vi "DailyReportSelectFromDateToDate.vi"() -> ()   [LabVIEW 2012]
uses:
  <vilib>/Utility/NIReport.llb/NI_report.lvclass
  Global1.vi
  <vilib>/Utility/NIReport.llb/Append Text Table to Report (wrap).vi
  <vilib>/Utility/NIReport.llb/Excel/NI_Excel.lvclass
  <vilib>/addons/_office/NI_ReportGenerationToolkit.lvlib
panel:
  in  "OK Button":bool
  in  "stop":bool
  in  "From Date (起日)":string="2014/9/20"
  in  "End Date (ùら)":string="2014/9/24"
  out "error out":errorcluster
  in  "ShiftB":string[][](array[string])
  in  "ShiftA":string[][](array[string])
  in  "ShiftC":string[][](array[string])
  in  "Summary":string[][](array[string])
  out "Row Headers":string[](array[string])
  in  "MonthToDate":string[][](array[string])
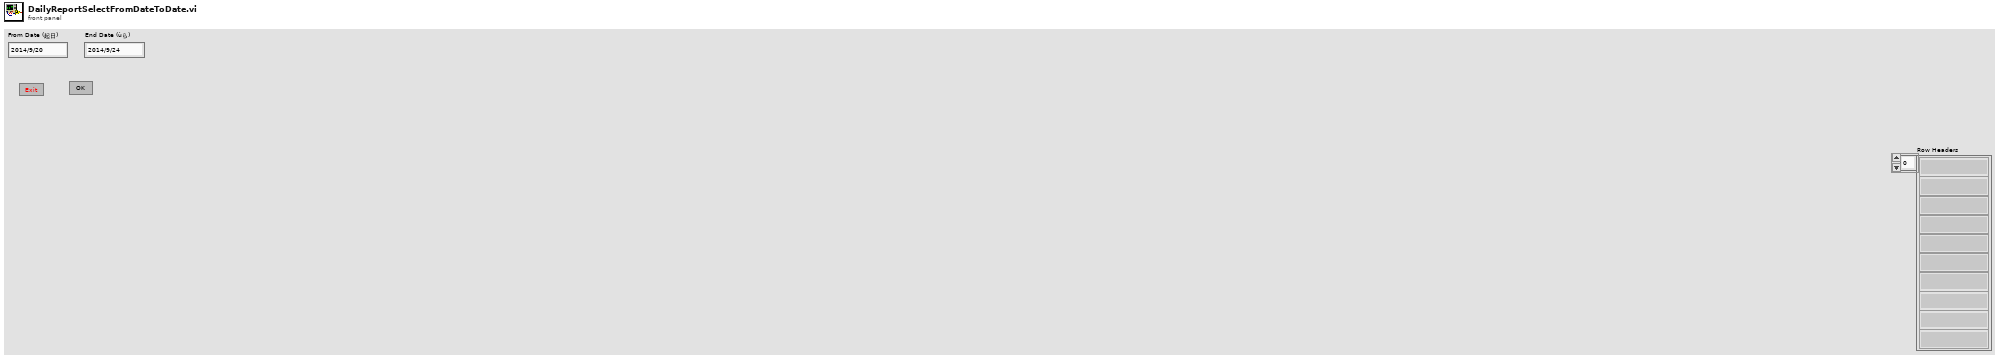
[diagram p1: front panel]
types:
  T1 = enum16{"Standard Report", "HTML", "Word", "Excel"}
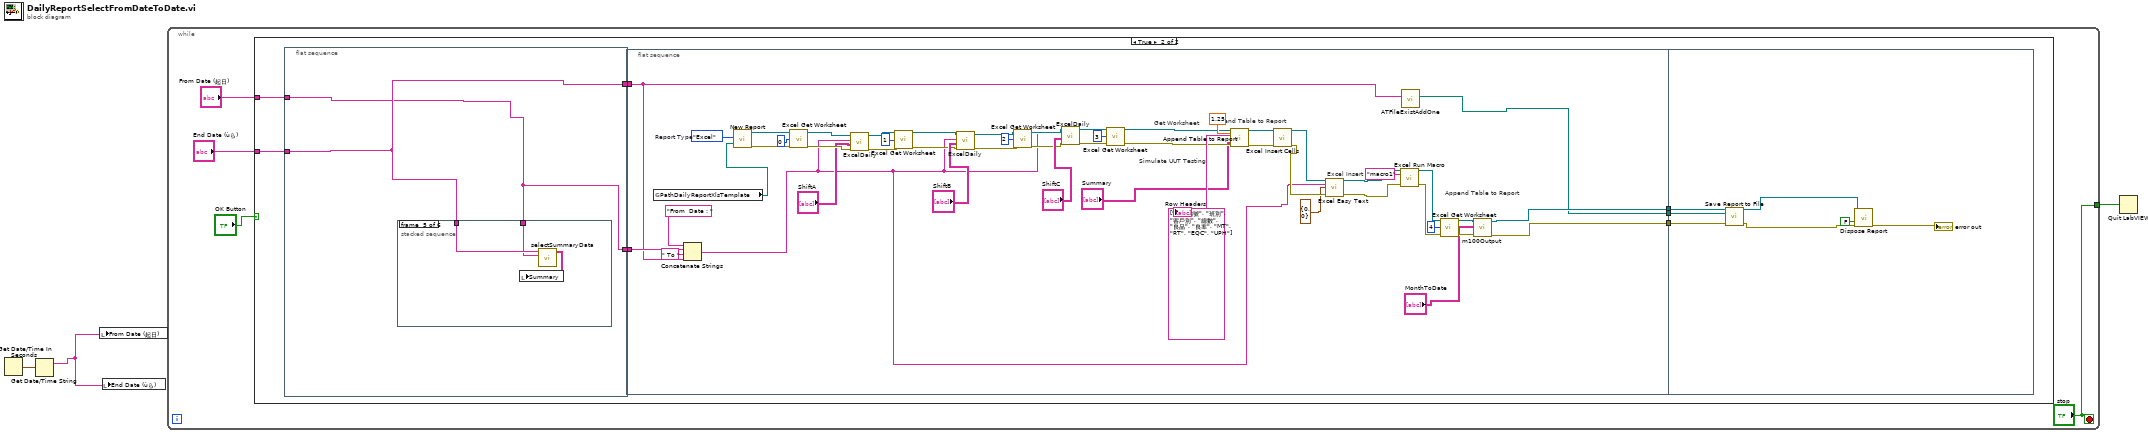
[diagram p0: block diagram]
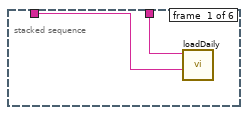
[diagram p3: hidden frame]
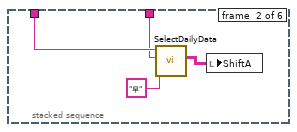
[diagram p4: hidden frame]
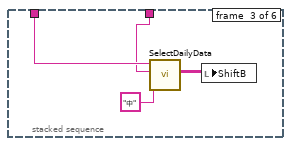
[diagram p5: hidden frame]
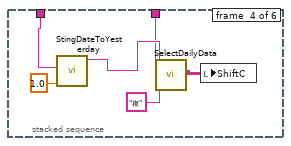
[diagram p6: hidden frame]
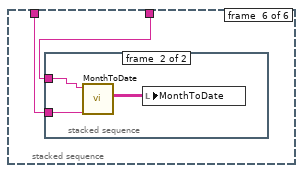
[diagram p7: hidden frame]
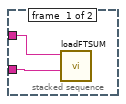
[diagram p8: hidden frame]
diagram:
  n1 = Get Date/Time In Seconds() -> (seconds since 1Jan1904=w3:timestamp)
  n2 = Get Date/Time String(seconds (now)=w3) -> (date string=w2:string)  [unwired: 2 in, 1 out]
  n3 = local write "From Date (起日)"(w2) -> ()
  n4 = local write "End Date (ùら)"(w2) -> ()
  n5 = while {
    tunnel: ["stop"] -> w1
    stop <- "stop" stop-if-true
    n6 = case shown="True" "OK Button" {
      tunnel: "From Date (起日)" -> [_ w10]
      tunnel: "End Date (ùら)" -> [_ w9]
      frame False {
      }
      frame True {
        n7 = flat-sequence {
          tunnel: [w73] -> w11
          tunnel: w10 -> [w72]
          tunnel: w9 -> [w73]
          tunnel: [w72] -> w8
          frame #0 {
            n8 = stacked-sequence {
              tunnel: w72 -> [w74 w76 w80 w84 w90 w93]
              tunnel: w73 -> [w75 w77 w81 w87 w91 w94]
              frame #0 {
                n9 = call "loadDaily.vi"("end date"=w75, "begin date"=w74) -> ()  [unwired: 9 in, 1 out]
              }
              frame #1 {
                n10 = call "SelectDailyData.vi"("Shift"="早", "Begin_date"=w76, "End_date"=w77) -> ("output array"=w78:string[][])  [unwired: 8 in]
                n11 = local write "ShiftA"(w78) -> ()
              }
              frame #2 {
                n12 = call "SelectDailyData.vi"("Shift"="中", "Begin_date"=w80, "End_date"=w81) -> ("output array"=w82:string[][])  [unwired: 8 in]
                n13 = local write "ShiftB"(w82) -> ()
              }
              frame #3 {
                n14 = call "StingDateToYesterday.vi"("Days"=1.0, "Date"=w87) -> ("Date+1"=w85:string)  [unwired: 8 in, 1 out]
                n15 = call "SelectDailyData.vi"("Shift"="夜", "Begin_date"=w84, "End_date"=w85) -> ("output array"=w88:string[][])  [unwired: 8 in]
                n16 = local write "ShiftC"(w88) -> ()
              }
              frame #4 {
                n17 = call "selectSummaryData.vi"("End Date"=w90, "From Date"=w91) -> ("Summary"=w92:string[][])  [unwired: 9 in]
                n18 = local write "Summary"(w92) -> ()
              }
              frame #5 {
                n19 = stacked-sequence {
                  tunnel: w94 -> [w96 w97]
                  tunnel: w93 -> [w95 w98]
                  frame #0 {
                    n20 = call "loadFTSUM.vi"("End Date"=w96, "From Date"=w95) -> ()  [unwired: 9 in, 1 out]
                  }
                  frame #1 {
                    n21 = call "MonthToDate.vi"("End Date"=w97, "From Date"=w98) -> ("output array"=w99:string[][])  [unwired: 8 in, 1 out]
                    n22 = local write "MonthToDate"(w99) -> ()
                  }
                }
              }
            }
          }
        }
        n23 = flat-sequence {
          tunnel: w11 -> [w17]
          tunnel: [w23] -> w14
          tunnel: [w22] -> w13
          tunnel: [w21] -> w12
          tunnel: w8 -> [w18]
          tunnel: w14 -> [w71]
          tunnel: w13 -> [w70]
          tunnel: w12 -> [w69]
          frame #0 {
            w42 = string[] ["機台編號", "班別", "客戶別", "總數", "良品", "良率", "MT", "RT", "EQC", "UPH"] ("row headers")
            w64 = T1."Excel"  # Report Type
            # "Append Table to Report"
            # "Excel Insert Text"
            # "Simulate UUT Testing"
            # "Append Table to Report"
            # "Get Worksheet"
            n24 = global read "Global1.vi" "PathDailyReportXlsTemplate"() -> (w24:path)
            n25 = Concatenate Strings("From  Date : " ("string"), w18, " To " ("string"), w17) -> (w15:string)
            n26 = call <vilib>:"New Report.vi"("report type"=w64, "template (empty)"=w24) -> ("report out"=w63:refnum<class "NI_report.lvclass">, "error out"=w62:errorcluster)  [unwired: 12 in]
            n27 = call <vilib>:"Excel Get Worksheet.vi"("report in"=w63, "worksheet index (0)"=0, "error in (no error)"=w62) -> ("report out"=w60:refnum<class "NI_report.lvclass">, "error out"=w59:errorcluster)  [unwired: 11 in]
            n28 = call "ExcelDaily.vi"("error in (no error)"=w59, "Input"="ShiftA", "Header"=w15, "report in"=w60) -> ("error out"=w53:errorcluster, "report out"=w55:refnum<class "NI_report.lvclass">)  [unwired: 6 in]
            n29 = call <vilib>:"Excel Get Worksheet.vi"("report in"=w55, "worksheet index (0)"=1, "error in (no error)"=w53) -> ("report out"=w54:refnum<class "NI_report.lvclass">, "error out"=w52:errorcluster)  [unwired: 11 in]
            n30 = call "ExcelDaily.vi"("error in (no error)"=w52, "Input"="ShiftB", "Header"=w15, "report in"=w54) -> ("error out"=w49:errorcluster, "report out"=w50:refnum<class "NI_report.lvclass">)  [unwired: 6 in]
            n31 = call <vilib>:"Excel Get Worksheet.vi"("report in"=w50, "worksheet index (0)"=2, "error in (no error)"=w49) -> ("report out"=w48:refnum<class "NI_report.lvclass">, "error out"=w16:errorcluster)  [unwired: 11 in]
            n32 = call "ExcelDaily.vi"("error in (no error)"=w16, "Input"="ShiftC", "Header"=w15, "report in"=w48) -> ("error out"=w45:errorcluster, "report out"=w46:refnum<class "NI_report.lvclass">)  [unwired: 6 in]
            n33 = call <vilib>:"Excel Get Worksheet.vi"("report in"=w46, "worksheet index (0)"=3, "error in (no error)"=w45) -> ("report out"=w33:refnum<class "NI_report.lvclass">, "error out"=w32:errorcluster)  [unwired: 11 in]
            n34 = call-poly <vilib>:"Append Table to Report.vi"("report in"=w33, "column width (1)"=1.25, "column headers"=w42, "text data"="Summary", "error in (no error)"=w32) -> ("report out"=w41:refnum<class "NI_report.lvclass">, "error out"=w40:errorcluster)  [unwired: 7 in, 2 out]
            n35 = call <vilib>:"Excel Insert Cells.vi"("report in"=w41, "error in (no error)"=w40) -> ("report out"=w39:refnum<class "NI_report.lvclass">, "error out"=w38:errorcluster)  [unwired: 12 in]
            n36 = call <vilib>:"Excel Easy Text.vi"("report in"=w39, "text"=w15, "start (-1, -1)"=cluster{"row":i32, "column":i32} {"row"=0, "column"=0} ("end (-1, -1)"), "error in (no error)"=w38) -> ("report out"=w36:refnum<class "NI_report.lvclass">, "error out"=w35:errorcluster)  [unwired: 7 in, 3 out]
            n37 = call <vilib>:"Excel Run Macro.vi"("report in"=w36, "macro name"="macro1", "error in (no error)"=w35) -> ("report out"=w30:refnum<class "NI_report.lvclass">, "error out"=w29:errorcluster)  [unwired: 10 in, 1 out]
            n38 = call "ATFileExistAddOne.vi"("input string"=w17) -> ("appended path"=w21:path)  [unwired: 10 in]
            n39 = call <vilib>:"Excel Get Worksheet.vi"("report in"=w30, "worksheet index (0)"=4, "error in (no error)"=w29) -> ("report out"=w27:refnum<class "NI_report.lvclass">, "error out"=w26:errorcluster)  [unwired: 11 in]
            n40 = call "m100Output.vi"("error in (no error)"=w26, "Input"="MonthToDate", "report in"=w27) -> ("error out"=w22:errorcluster, "report out"=w23:refnum<class "NI_report.lvclass">)  [unwired: 7 in]
            "Row Headers" <- w42
          }
          frame #1 {
            n41 = call-dynamic "Save Report to File.vi"("report in"=w71, "report file path"=w69, "error in (no error)"=w70) -> ("report out"=w68:refnum<class "NI_report.lvclass">, "error out"=w67:errorcluster)  [unwired: 11 in]
            n42 = call-dynamic "Dispose Report.vi"("report in"=w68, "save changes? (F)"=FALSE, "error in (no error)"=w67) -> ("error out"=→"error out":errorcluster)  [unwired: 12 in]
          }
        }
      }
    }
  }
  n43 = Quit LabVIEW(quit? (T)=w1) -> ()
